vi "PH_PSDBWriter.declare Proc Events.vi"() -> (0 "PSDB DIM Service Events":T1[](array[typedef]))   [LabVIEW 2014, in "PH_PSDBWriter.lvlib"]
doc: "within this VI the proc events of the proc cases of the PSDB Writer are declared (if the PSDB-Controller is not N/A or empty)."
uses:
  PH_PSDBWriter.lvlib
  CS_Core/BaseProcess/BaseProcess.event definition.ctl
  CS_Core/CAEObj/CAEObj.event definition.ctl
  CS_Core/BaseProcess/BaseProcess.descriptor string definition.ctl
  CS_Core/BaseProcess/BaseProcess.lvlib
  CS_Core/CAEObj/CAEObj.lvlib
  PH_Common/PH_Common.lvlib
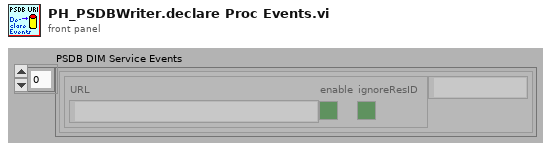
[diagram p1: front panel]
types:
  T1 = typedef "BaseProcess.lvlib/BaseProcess.event definition.ctl" = cluster{"CAEEvtDef":T2, "Data Descriptor":T3}
  T2 = typedef "CAEObj.lvlib/CAEObj.event definition.ctl" = cluster{"URL":string, "enable":bool, "ignoreResID":bool}
  T3 = typedef "BaseProcess.lvlib/BaseProcess.descriptor string definition.ctl" = string
  T4 = typedef "PH_Common.lvlib/PH_DIM.Event Declarer.ctl" = cluster{"Service Name":string, "Selector":string}
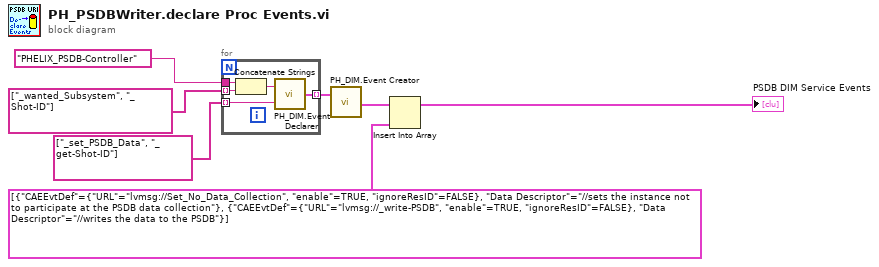
[diagram p0: block diagram]
diagram:
  n1 = for {
    tunnel: [w10] -> w3 mode=indexing
    tunnel: string[] ["_set_PSDB_Data", "_get-Shot-ID"] -> [w8] mode=indexing
    tunnel: string[] ["_wanted_Subsystem", "_Shot-ID"] -> [w11] mode=indexing
    tunnel: "PHELIX_PSDB-Controller" ("PSDB Controller") -> [w12]
    n2 = Concatenate Strings(w12, w11) -> (w9:string)
    n3 = call "PH_DIM.Event Declarer.vi"("Selector"=w8, "Service Name"=w9) -> ("declared DIM Event"=w10:T4)
  }
  n4 = call "PH_DIM.Event Creator.vi"("Trendmessage Services"=w3) -> ("DIM Service Events"=w2:T1[])  [unwired: 18 in]
  n5 = Insert Into Array(array=w2, new element=T1[] [{"CAEEvtDef"={"URL"="lvmsg://Set_No_Data_Collection", "enable"=TRUE, "ignoreResID"=FALSE}, "Data Descriptor"="//sets the instance not to participate at the PSDB data collection"}, {"CAEEvtDef"={"URL"="lvmsg://_write-PSDB", "enable"=TRUE, "ignoreResID"=FALSE}, "Data Descriptor"="//writes the data to the PSDB"}] ("new events")) -> (→"PSDB DIM Service Events":T1[])  [unwired: 1 in]
